vi "WPI_GyroOpen.vi"(6 "Calibrated Center Voltage":dbl, 7 "Calibration Time (s)":dbl=2.0, 8 "error in (no error)":errorcluster, 9 "Calibrate On Open":bool=TRUE, 10 "Analog Channel":T2, 11 "Analog Module (Module 1)":T1) -> (0 "error out":errorcluster, 2 "Calibrated Center Voltage Out":dbl, 3 "GyroDevRef":T3)   [LabVIEW 2013]
doc: "Opens a reference to the gyroscope you specify. You must open a reference before using any other VIs on this palette.\n\nThis software is licensed. Open the labview\\readme\\WPI Robotics Library Open Source License.txt file for more information."
uses:
  <vilib>/Rock Robotics/WPI/Gyro/WPI_GyroDevRef.ctl
  <vilib>/Rock Robotics/SystemInterfaces/Typedef/FPGA_TypedefAnalogModule.ctl
  <vilib>/Rock Robotics/SystemInterfaces/AI/FPGA_AIChannel.ctl
  <vilib>/Rock Robotics/SystemInterfaces/AI/FPGA_AIGyroChannel.ctl
  <vilib>/Rock Robotics/SystemInterfaces/Typedef/FPGA_TypedefAnalogModuleForGyro.ctl
  <vilib>/robotics/Simulator/Engine/ctl/DeviceID.ctl
  <instrlib>/Sparkfun Atomic IMU/HAIOL/Simulator/Sparkfun Atomic IMU Simulator.lvclass
  <vilib>/robotics/Simulator/NI_Robotics_Simulator.lvlib
  <instrlib>/Honeywell Compass HMC6343/HAIOL/Simulator/Honeywell Compass HMC6343 Simulator.lvclass
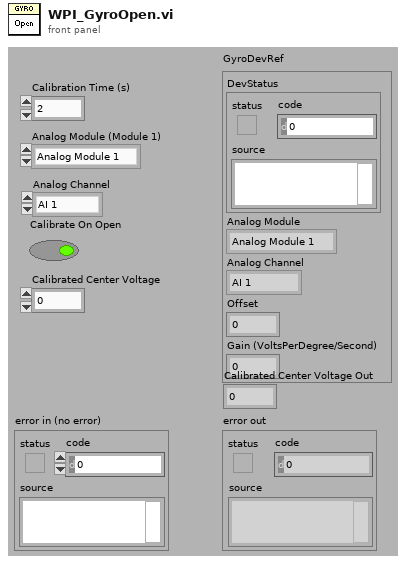
[diagram p1: front panel]
types:
  T1 = typedef "FPGA_TypedefAnalogModuleForGyro.ctl" = enum16{"Analog Module 1"}
  T2 = typedef "FPGA_AIGyroChannel.ctl" = enum8{"AI 1", "AI 2", "Invalid"}
  T3 = typedef "WPI_GyroDevRef.ctl" = cluster{"DevStatus":errorcluster, "Analog Module":T4, "Analog Channel":T5, "Offset":dbl, "Gain (VoltsPerDegree/Second)":dbl}
  T4 = typedef "FPGA_TypedefAnalogModule.ctl" = enum16{"Analog Module 1", "Analog Module 2"}
  T5 = typedef "FPGA_AIChannel.ctl" = enum8{"AI 1", "AI 2", "AI 3", "AI 4", "AI 5", "AI 6", "AI 7", "AI 8", "Invalid"}
  T6 = typedef "NI_Robotics_Simulator.lvlib/DeviceID.ctl" = cluster{"robot ID":string, "sensor/actuator ID":string}
  T7 = typedef "WPI_AnalogChannelDevRef.ctl" = cluster{"DevStatus":errorcluster, "Analog Module":T4, "Analog Channel":T5}
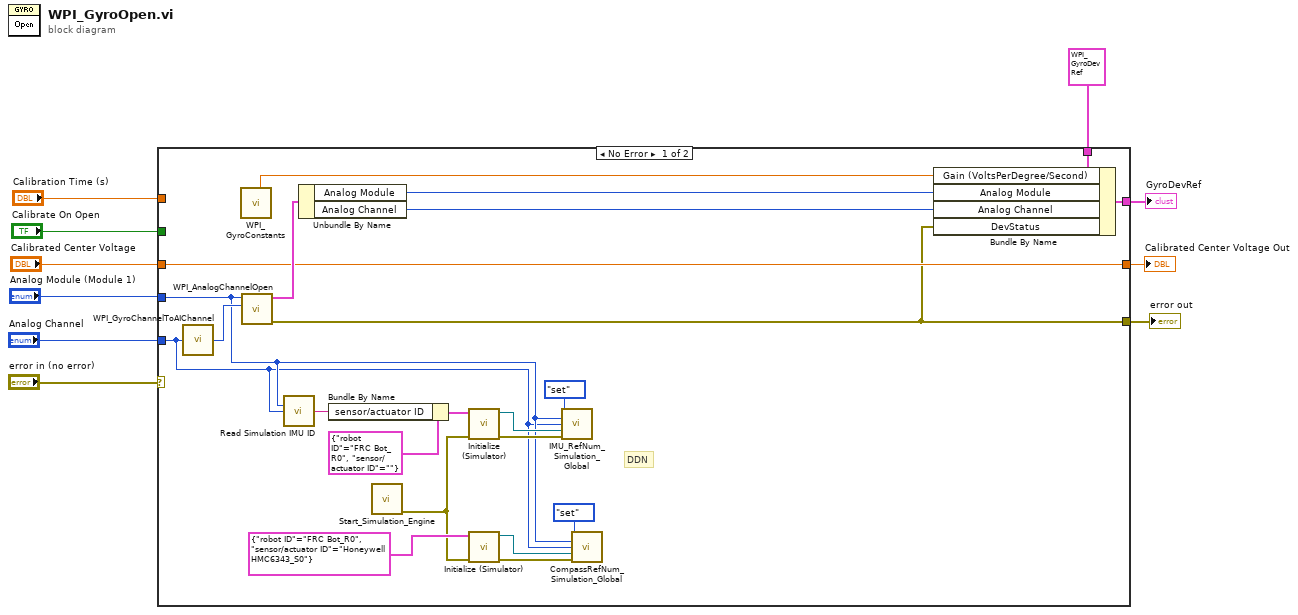
[diagram p0: block diagram]
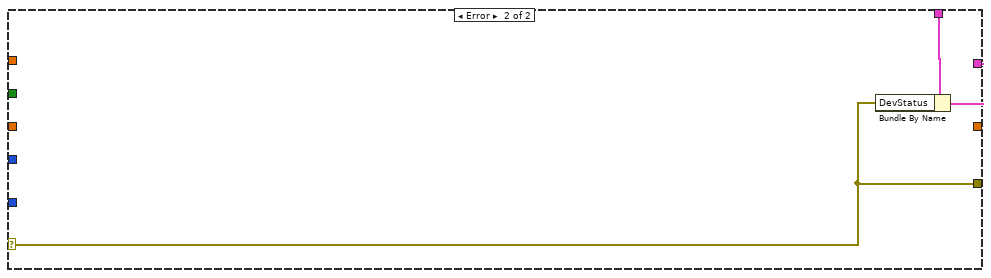
[diagram p2: hidden frame]
diagram:
  n1 = case shown="No Error" "error in (no error)" {
    selector: "error in (no error)" -> [_ w33]
    tunnel: "Analog Module (Module 1)" -> [w17 _]
    tunnel: "Analog Channel" -> [w16 _]
    tunnel: [w24 w33] -> w9
    tunnel: T3 {"DevStatus"={"status"=FALSE, "code"=0, "source"=""}, "Analog Module"=enum."Analog Module 1", "Analog Channel"=enum."Invalid", "Offset"=0.0, "Gain (VoltsPerDegree/Second)"=0.0} ("GryoDevStatus") -> [w30 w34]
    tunnel: [w29 w35] -> w6
    tunnel: "Calibrate On Open" -> [_ _]
    tunnel: "Calibrated Center Voltage" -> [w25 _]
    tunnel: "Calibration Time (s)" -> [_ _]
    tunnel: [w25 _] -> w1
    frame No Error {
      # "DDN"
      n2 = call "WPI_GyroChannelToAIChannel.vi"("Gyro Channel"=w16) -> ("AI Channel"=w28:T5)  [unwired: 4 out]
      n3 = call "WPI_GyroConstants.vi"() -> ("Gain (VoltsPerDegreePerSecond)"=w26:dbl)  [unwired: 11 out]
      n4 = call <vilib>:"WPI_AnalogChannelOpen.vi"("Analog Channel"=w28, "Analog Module (Module 1)"=w17) -> ("error out"=w24:errorcluster, "AIDeviceRef"=w27:T7)  [unwired: 1 in, 7 out]
      n5 = call <vilib>:"Read Simulation IMU ID.vi"("Analog Module (Module 1)"=w17, "Analog Channel"=w16) -> ("gyro ID"=w21:string)  [unwired: 12 in, 1 out]
      n6 = Unbundle By Name(w27) -> ("Analog Module"=w32:T4, "Analog Channel"=w31:T5)
      n7 = Bundle By Name(cluster=T6 {"robot ID"="FRC Bot_R0", "sensor/actuator ID"=""} ("Device ID"), "sensor/actuator ID"=w21) -> (w22:T6)
      n8 = call <vilib>:"Start_Simulation_Engine.vi"() -> ("error out"=w14:errorcluster)  [unwired: 15 in]
      n9 = call <instrlib>:"Initialize (Simulator).vi"("error in (no error)"=w14, "Device ID"=w22) -> ("error out"=w18:errorcluster, "Sparkfun Atomic IMU out"=w20:refnum<class "Sparkfun Atomic IMU.lvclass">)  [unwired: 8 in]
      n10 = call <instrlib>:"Initialize (Simulator).vi"("error in (no error)"=w14, "Device ID"=T6 {"robot ID"="FRC Bot_R0", "sensor/actuator ID"="Honeywell HMC6343_S0"}) -> ("error out"=w12:errorcluster, "Honeywell Compass HMC6343"=w11:refnum<class "Honeywell Compass HMC6343.lvclass">)  [unwired: 8 in]
      n11 = call <vilib>:"IMU_RefNum_Simulation_Global.vi"("menu"=enum16{"set", "get", "delete"}."set", "Analog Module (Module 1)"=w17, "Analog Channel"=w16, "Sparkfun Atomic IMU Set"=w20, "error in (no error)"=w18) -> ()  [unwired: 9 in, 2 out]
      n12 = call <vilib>:"CompassRefNum_Simulation_Global.vi"("menu"=enum16{"set", "get", "delete"}."set", "Analog Module (Module 1)"=w17, "Analog Channel"=w16, "Honeywell Compass HMC6343 Set"=w11, "error in (no error)"=w12) -> ()  [unwired: 9 in, 2 out]
      n13 = Bundle By Name(cluster=w30, "Gain (VoltsPerDegree/Second)"=w26, "Analog Module"=w32, "Analog Channel"=w31, "DevStatus"=w24) -> (w29:T3)
    }
    frame Error {
      n14 = Bundle By Name(cluster=w34, "DevStatus"=w33) -> (w35:T3)
    }
  }
  "GyroDevRef" <- w6
  "error out" <- w9
  "Calibrated Center Voltage Out" <- w1
